vi "Buffer.vi"() -> ()   [LabVIEW 2013]
panel:
  in  "IDN?":string
  in  "new?":bool=TRUE
  in  "Detail":string
  in  "ReadBuffer":string
  in  "HPT OPID":string
  in  "CheckSN":bool=TRUE
  in  "MAIN_Ver":string
  in  "Outside OPID":string
  in  "OPID":string
  out "testlist":dbl[](array[numeric])
  in  "Password":string
  in  "Continue":string="T"
  in  "Station":string="TEST"
  in  "Disk":string="C:\\"
  in  "AutoModel":bool
  out "ledc":bool=TRUE
  in  "LabelSN":string="111111111111111111111111111"
  in  "MonitorScanner?":bool
  in  "TrigerNO.":i32=64
  in  "Triger Not?":bool
  in  "CallGeaWay":bool=TRUE
  in  "STOP ROW":i32
  in  "Model":string="GEA"
  in  "PSU":string="245D1776G001"
  in  "Barcode(SN)length":string="27"
  in  "Barcode(SN)offset":string="0"
  in  "Triger":bool=TRUE
  in  "SN":string
  in  "Debug":bool=TRUE
  in  "Steps":i32=11
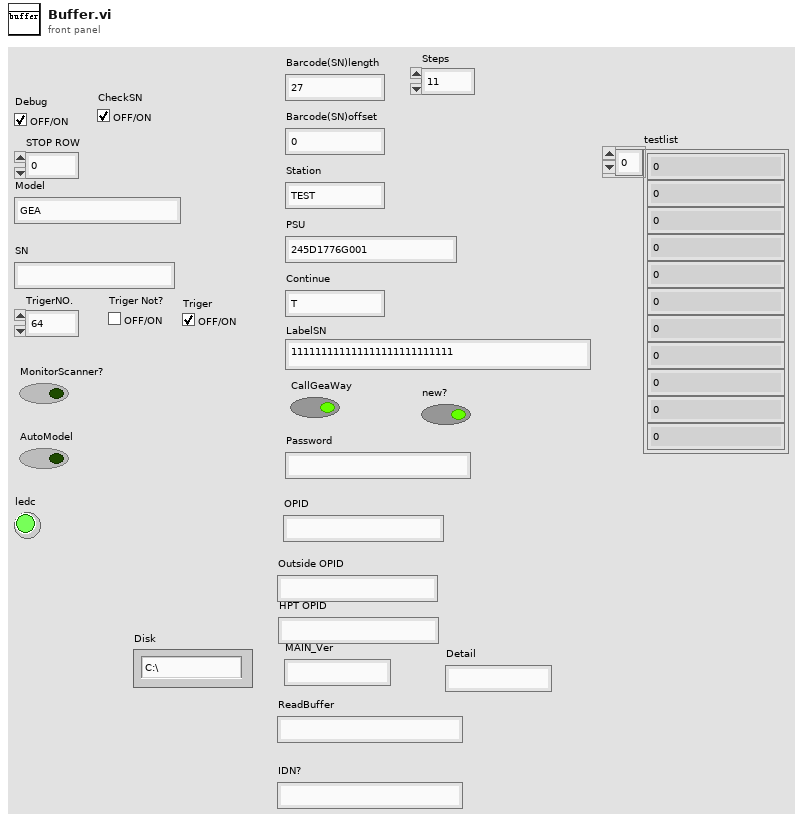
[diagram p1: front panel]
diagram:
